vi "Setpoint Status.vi"(8 "error in (no error)":errorcluster, 10 "Loop (1:Loop 1)":u16(ring)=1 items=["Loop 1"=1, "Loop 2"=2], 11 "VISA resource name":refnum<visa-resource-name>) -> (0 "error out":errorcluster, 2 "Setpoint Value":dbl format="%.4f", 3 "VISA resource name out":refnum<visa-resource-name>)   [LabVIEW 2019, in "Lake Shore 325.lvlib"]
doc: "This VI returns the control setpoint value. The control setpoint is the desired load temperature expressed in temperature or sensor units."
uses:
  <instrlib>/Lake Shore 325/Lake Shore 325.lvlib
  Instance           1 23Saved   Setpoint Status .vi
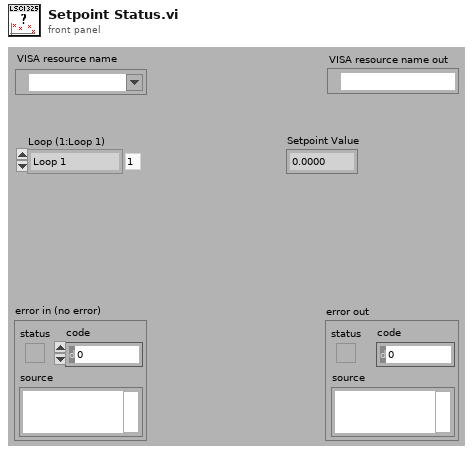
[diagram p1: front panel]
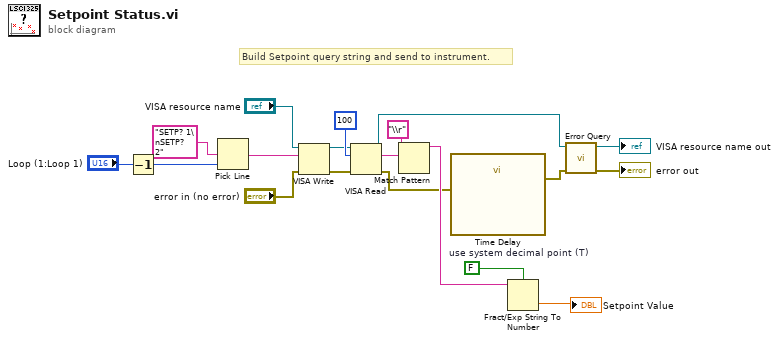
[diagram p0: block diagram]
diagram:
  w6 = FALSE  # use system decimal point (T)
  # "Build Setpoint query string and send to instrument."
  n1 = Decrement(x="Loop (1:Loop 1)") -> (x-1=w12:u16)
  n2 = Pick Line(multi-line string="SETP? 1\nSETP? 2", line index=w12) -> (output string=w4:string)  [unwired: 1 in]
  n3 = VISA Write(VISA resource name="VISA resource name", write buffer=w4, error in (no error)="error in (no error)") -> (VISA resource name out=w8:refnum<visa-resource-name>, error out=w7:errorcluster)  [unwired: 1 out]
  n4 = VISA Read(VISA resource name=w8, byte count=100, error in (no error)=w7) -> (VISA resource name out=w15:refnum<visa-resource-name>, read buffer=w10:string, error out=w1:errorcluster)  [unwired: 1 out]
  n5 = Match Pattern(string=w10, regular expression="\\r") -> (before substring=w3:string)  [unwired: 1 in, 3 out]
  n6 = call "Time Delay"("error in (no error)"=w1) -> ("error out"=w2:errorcluster)  [unwired: 10 in]
  n7 = Fract/Exp String To Number(use system decimal point (T)=w6, string=w3) -> (number=→"Setpoint Value":dbl)  [unwired: 2 in, 1 out]
  n8 = call <instrlib>:"Error Query.vi"("error in (no error)"=w2, "VISA resource name"=w15) -> ("error out"=→"error out":errorcluster, "VISA resource name out"=→"VISA resource name out":refnum<visa-resource-name>)  [unwired: 7 in, 1 out]
